vi "subXMLGetDestinationDir.vi"(9 "Project path":path, 11 "Refnum in":refnum<k20>) -> (1 "Name":string, 3 "Path":path)   [LabVIEW 2019, in "SolutionBuilder.lvlib" / "SolutionBuilder.lvclass"]
uses:
  SolutionBuilder.lvclass
  <vilib>/xml/NI_XML.lvlib
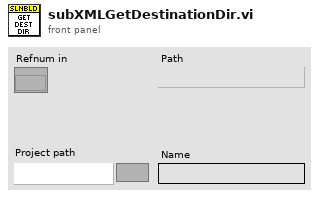
[diagram p1: front panel]
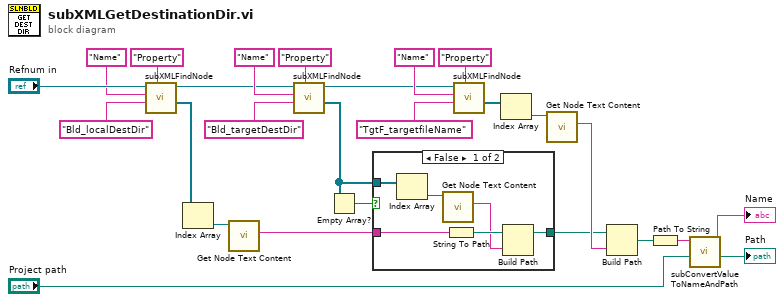
[diagram p0: block diagram]
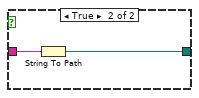
[diagram p2: hidden frame]
diagram:
  n1 = call "subXMLFindNode.vi"("Node name"="Property", "Property value"="Bld_localDestDir", "Property name"="Name", "Refnum in"="Refnum in") -> ("Nodes"=w24:refnum<k20>[], "Refnum"=w6:refnum<k20>)  [unwired: 6 in]
  n2 = Index Array(array=w24) -> (element=w25:refnum<k20>)  [unwired: 1 in]
  n3 = call <vilib>:"Get Node Text Content.vi"("node in"=w25) -> ("node text"=w2:string)  [unwired: 8 in, 2 out]
  n4 = call "subXMLFindNode.vi"("Node name"="Property", "Property value"="Bld_targetDestDir", "Property name"="Name", "Refnum in"=w6) -> ("Nodes"=w4:refnum<k20>[], "Refnum"=w5:refnum<k20>)  [unwired: 6 in]
  n5 = Empty Array?(array=w4) -> (empty?=w3:bool)
  n6 = case shown="False" w3 {
    tunnel: w4 -> [w31 _]
    tunnel: w2 -> [w29 w34]
    tunnel: [w27 w33] -> w1
    frame False {
      n7 = Index Array(array=w31) -> (element=w32:refnum<k20>)  [unwired: 1 in]
      n8 = call <vilib>:"Get Node Text Content.vi"("node in"=w32) -> ("node text"=w28:string)  [unwired: 8 in, 2 out]
      n9 = String To Path(string=w29) -> (path=w30:path)
      n10 = Build Path(base path=w30, name or relative path=w28) -> (appended path=w27:path)
    }
    frame True {
      n11 = String To Path(string=w34) -> (path=w33:path)
    }
  }
  n12 = call "subXMLFindNode.vi"("Node name"="Property", "Property value"="TgtF_targetfileName", "Property name"="Name", "Refnum in"=w5) -> ("Nodes"=w15:refnum<k20>[])  [unwired: 6 in, 1 out]
  n13 = Index Array(array=w15) -> (element=w14:refnum<k20>)  [unwired: 1 in]
  n14 = call <vilib>:"Get Node Text Content.vi"("node in"=w14) -> ("node text"=w12:string)  [unwired: 8 in, 2 out]
  n15 = Build Path(base path=w1, name or relative path=w12) -> (appended path=w11:path)
  n16 = Path To String(path=w11) -> (string=w10:string)
  n17 = call "subConvertValueToNameAndPath.vi"("Project path"="Project path", "Value"=w10) -> ("Path"=→"Path":path, "Name"=→"Name":string)  [unwired: 8 in]
